vi "VRM.Clamp.vi"(6 "Axis":T1=enum."Z", 8 "error in (no error)":errorcluster, 11 "Instrument.VRM in":refnum<class "Instrument.OxfordVRM.lvclass">) -> (0 "error out":errorcluster, 2 "Response":string[](array[string]), 3 "Instrument.VRM out":refnum<class "Instrument.OxfordVRM.lvclass">)   [LabVIEW 2019, in "Instrument.OxfordVRM.lvclass"]
uses:
  Instrument.OxfordVRM.lvclass
  Typedefs/VRM Magnet Axis--Enum.ctl
  <instrlib>/Mercury iXX/Public/Libraries/Magnet/Controls/PSU Actions.ctl
  <instrlib>/Mercury iXX/Public/Libraries/Magnet.lvlib
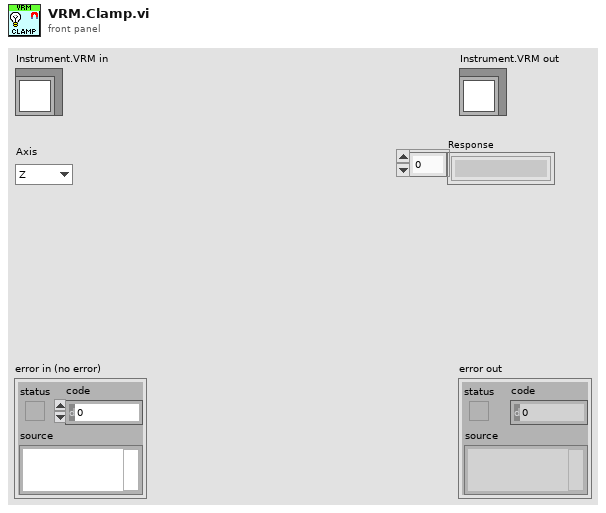
[diagram p1: front panel]
types:
  T1 = typedef "Instrument.OxfordVRM.lvclass/VRM Magnet Axis--Enum.ctl" = enum16{"X", "Y", "Z", "ALL"}
  T2 = typedef "Mercury iXX.lvlib/Magnet.lvlib/PSU Actions.ctl" = string
  T3 = typedef "Instrument.Cryostat.lvclass/Magnet Axis--Enum.ctl" = enum16{"X", "Y", "Z"}
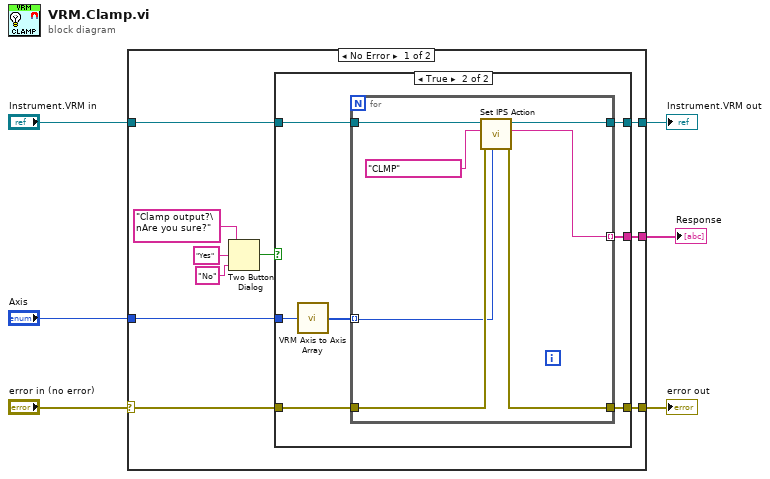
[diagram p0: block diagram]
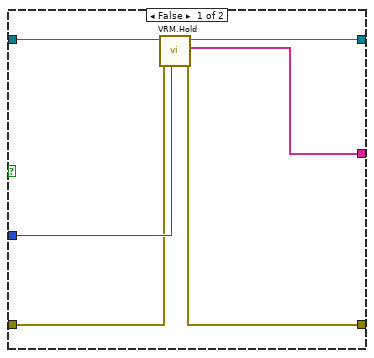
[diagram p2: hidden frame]
diagram:
  n1 = case shown="No Error" "error in (no error)" {
    selector: "error in (no error)" -> [w15 w38]
    tunnel: [w13 w38] -> w5
    tunnel: [w14 w37] -> w3
    tunnel: "Instrument.VRM in" -> [w16 w37]
    tunnel: "Axis" -> [w12 _]
    tunnel: [w7 _] -> w1
    frame No Error {
      n2 = Two Button Dialog(message="Clamp output?\nAre you sure?", 1:"No" ("F button name (\"Cancel\")"), 2:"Yes" ("T button name (\"OK\")")) -> (T button?=w8:bool)
      n3 = case shown="True" w8 {
        tunnel: w16 -> [w21 w29]
        tunnel: w15 -> [w18 w28]
        tunnel: [w20 w27] -> w14
        tunnel: [w19 w26] -> w13
        tunnel: w12 -> [w22 w24]
        tunnel: [w17 w23] -> w7
        frame False {
          n4 = call "VRM.Hold.vi"("Axis"=w22, "error in (no error)"=w18, "Instrument.VRM in"=w21) -> ("error out"=w19:errorcluster, "Response"=w17:string[], "Instrument.VRM out"=w20:refnum<class "Instrument.OxfordVRM.lvclass">)  [unwired: 6 in]
        }
        frame True {
          n5 = call "VRM Axis to Axis Array.vi"("Axis"=w24) -> ("Axis Array"=w25:T3[])
          n6 = for {
            tunnel: w29 -> [w35]
            tunnel: [w33] -> w27
            tunnel: w28 -> [w34]
            tunnel: [w31] -> w26
            tunnel: w25 -> [w32] mode=indexing
            tunnel: [w30] -> w23 mode=indexing
            n7 = call "Set IPS Action.vi"("Axis"=w32, "error in (no error)"=w34, "PSU Act Stat"=T2 "CLMP", "Instrument.OxfordVRM in"=w35) -> ("error out"=w31:errorcluster, "Response"=w30:string, "Instrument.OxfordVRM out"=w33:refnum<class "Instrument.OxfordVRM.lvclass">)  [unwired: 5 in]
          }
        }
      }
    }
    frame Error {
    }
  }
  "error out" <- w5
  "Instrument.VRM out" <- w3
  "Response" <- w1
